vi "Double FFT Mesurament (Max Bin detection - Control - Windowing - LEO) test.vi"() -> ()   [LabVIEW 2014]
uses:
  <vilib>/Platform/TimedLoop/XDataNode/timing_clust.ctl
  <vilib>/Platform/TimedLoop/XDataNode/nitl_modes.ctl
  <vilib>/Platform/TimedLoop/XDataNode/wakeup.ctl
  <vilib>/rvi/Analysis/measure/FFT/simModelSupport/niFPGA FFT Streaming Sim Properties.ctl
  <vilib>/rvi/Analysis/measure/FFT/simModelSupport/niFPGA FFT Sim Stream Group Properties.ctl
  <vilib>/rvi/Analysis/measure/FFT/simModelSupport/niFPGA FFT Sim Types.ctl
  <vilib>/rvi/Analysis/measure/FFT/simModelSupport/niFpgaFFTSimArithmeticProperties.ctl
  <vilib>/rvi/Analysis/measure/FFT/simModelSupport/niFpgaFFTSimDfxp.ctl
  <vilib>/fxp/LVFixedPointQuantizationPolicyTypeDef.ctl
  <vilib>/rvi/Analysis/measure/FFT/XNode/niFpgaFFTButterflyDelays.ctl
  <vilib>/rvi/Emulation/niFpgaSctlEmulationGetInTimedLoop.vi
  <vilib>/rvi/Emulation/niFpgaEmulationReportErrorSimple.vi
  <vilib>/rvi/Emulation/niFpgaGetClockAttributes.vi
  <vilib>/rvi/Emulation/niFpgaCriticalErrorInLSC.vi
  <vilib>/rvi/Emulation/niFpgaEmulationIsFPGAContextNoSignature.vi
  <vilib>/rvi/errors/niFpgaSetErrorForExecOnDevCompSimple.vi
  <vilib>/rvi/eio/common/nirviEmuReportErrorAndStop.vi
  <vilib>/rvi/DataTransferAndStorage/Container/Common/niFpgaContainerGetUniqueNameForEmu.vi
  <vilib>/rvi/FIFO/Fifo_Resource/nirvififoEmulationSetSize.vi
  <vilib>/rvi/FIFO/Fifo_Resource/nirviFifoEmulationQueueMgr.vi
  <instcachedir>/0/nirviFifoEmulationQueueMgr_E5CAEC123FF24DC58D834DCA3CDAA9B5.lvgen/nirviFifoEmulationQueueMgr_E5CAEC123FF24DC58D834DCA3CDAA9B5_012.vi
  <vilib>/rvi/FIFO/Fifo_Resource/nirvififoEmulationCreateLock.vi
  <vilib>/rvi/Emulation/niFpgaProcessEmulError.vi
  <vilib>/rvi/FIFO/Fifo_Resource/nirvififoEmulationObtainLock.vi
  <vilib>/rvi/FIFO/Fifo_Resource/nirvififoEmulationReleaseLock.vi
  <vilib>/rvi/occurrence/nirviWaitOnOccurrenceBase.vi
  <vilib>/rvi/errors/nirviReportUnexpectedCaseInternalError.vi
  <vilib>/rvi/errors/nirviReportUnexpectedCaseInternalError (U32).vi
  <vilib>/rvi/Memory/Memory_Emulation/niFpgaMemoryEmulationCacheClearOnFirstRun.vi
  <vilib>/rvi/Memory/Memory_Emulation/nirvimemoryEmulationManagerCache_MakeExclusive.vi
  <vilib>/rvi/Memory/Memory_Emulation/niFpgaMemoryEmulationValidateCache.vi
  <vilib>/rvi/Memory/Memory_Emulation/nirvimemoryEmulationManagerCache_InsertValue.vi
  <vilib>/Utility/error.llb/Clear Errors.vi
  <vilib>/rvi/Memory/Memory_Emulation/nirvimemoryEmulationManagerCache_ReleaseExclusive.vi
  <vilib>/rvi/Memory/Memory_Emulation/nirvimemoryEmulationManagerCache_GetValue.vi
  <vilib>/rvi/Memory/Memory_Emulation/nirvimemoryEmulationManagerCache_SetValue.vi
  <vilib>/rvi/interface/RandomDataEmulation/niFpgaRandomDataHandleErrors.vi
  <instcachedir>/0/nirviFifoEmulationQueueMgr_E5CAEC123FF24DC58D834DCA3CDAA9B5.lvgen/nirviFifoEmulationQueueMgr_E5CAEC123FF24DC58D834DCA3CDAA9B5_010.vi
  <vilib>/rvi/FIFO/Fifo_Resource/nirvififoEmulationDetermineInputValidOut.vi
  <vilib>/rvi/Memory/Memory_Emulation/nirvimemoryFastEmulation.vi
  <vilib>/rvi/Memory/Memory_Emulation/nirvimemoryEmulation.vi
  <vilib>/rvi/Analysis/measure/FFT/simModelSupport/niFpgaFFTSimModelStreamingCore.vi
  <vilib>/rvi/eio/common/nirviEmuTemplateMethod_errors.vi
  <vilib>/Platform/TimedLoop/XDataNode/XDataNode.xnode
  <vilib>/rvi/DataTransferAndStorage/Container/XNode/niFpgaContainer.xnode
  <vilib>/rvi/FIFO/Fifo_Resource/nirvififoEmulationRead.vi
  <vilib>/rvi/DataTransferAndStorage/Register/Emulation/niFpgaRegisterEmulation.vi
  <vilib>/rvi/interface/RandomDataEmulation/nirviRandomDataFpgaReadWriteTemplate.vi
  <vilib>/rvi/FIFO/Fifo_Resource/nirvififoEmulationWrite.vi
  <vilib>/rvi/FIFO/Fifo_Resource/nirvififoEmulationGetNumberOfElementsToWrite.vi
  <vilib>/rvi/Analysis/measure/FFT/XNode/niFpgaFFT.xnode
  <vilib>/eio/EIOMethodNode/EIOMethodNode.xnode
  <vilib>/Platform/TimedLoop/XDataNode/XDNodeRunTimeDep.lvlib
panel:
  in  "first bin":i32=4
  in  "last bin":i32=251
  in  "lower limit 2":u32=682
  in  "lower limit 1":u32=57
  in  "upper limit 2":u32=1194
  in  "upper limit 1":u32=569
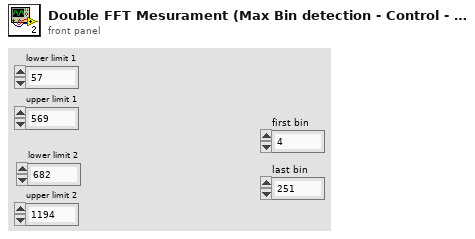
[diagram p1: front panel]
types:
  T1 = typedef "XDNodeRunTimeDep.lvlib/timing_clust.ctl" = cluster{"Expected End [f-1]":u64, "Actual End [f-1]":u64, "Finished Late? [f-1]":bool, "Expected End [i-1]":u64, "Actual End [i-1]":u64, "Finished Late? [i-1]":bool, "Expected Start [i]":u64, "Actual Start [i]":u64, "Expected Start [f]":u64, "Actual Start [f]":u64, "Source Name":string, "Structure Name":string, "Period":i64, "Deadline":i64, "Offset":i64, "Start":i64, "Priority":i32, "Timeout":i32, "Mode":T2, "Wakeup Reason":T3, "Error":errorcluster, "Source Type":string, "Secondary Source Type":string, "Global End Time":u64, "Global Start Time":u64, "Frame Duration":u64, "Iteration Duration":u64, "Assigned CPU":i32, "I/O Scan Engine Mode":u32}
  T2 = typedef "XDNodeRunTimeDep.lvlib/nitl_modes.ctl" = enum32{"No Change", "Process missed periods, maintain original phase", "Discard missed periods, maintain original phase", "Process missed periods, ignore original phase", "Discard missed periods, ignore original phase"}
  T3 = typedef "XDNodeRunTimeDep.lvlib/wakeup.ctl" = enum32{"Normal", "Aborted", "Asynchronous wakeup", "Timing source error", "Timed loop error", "Timeout"}
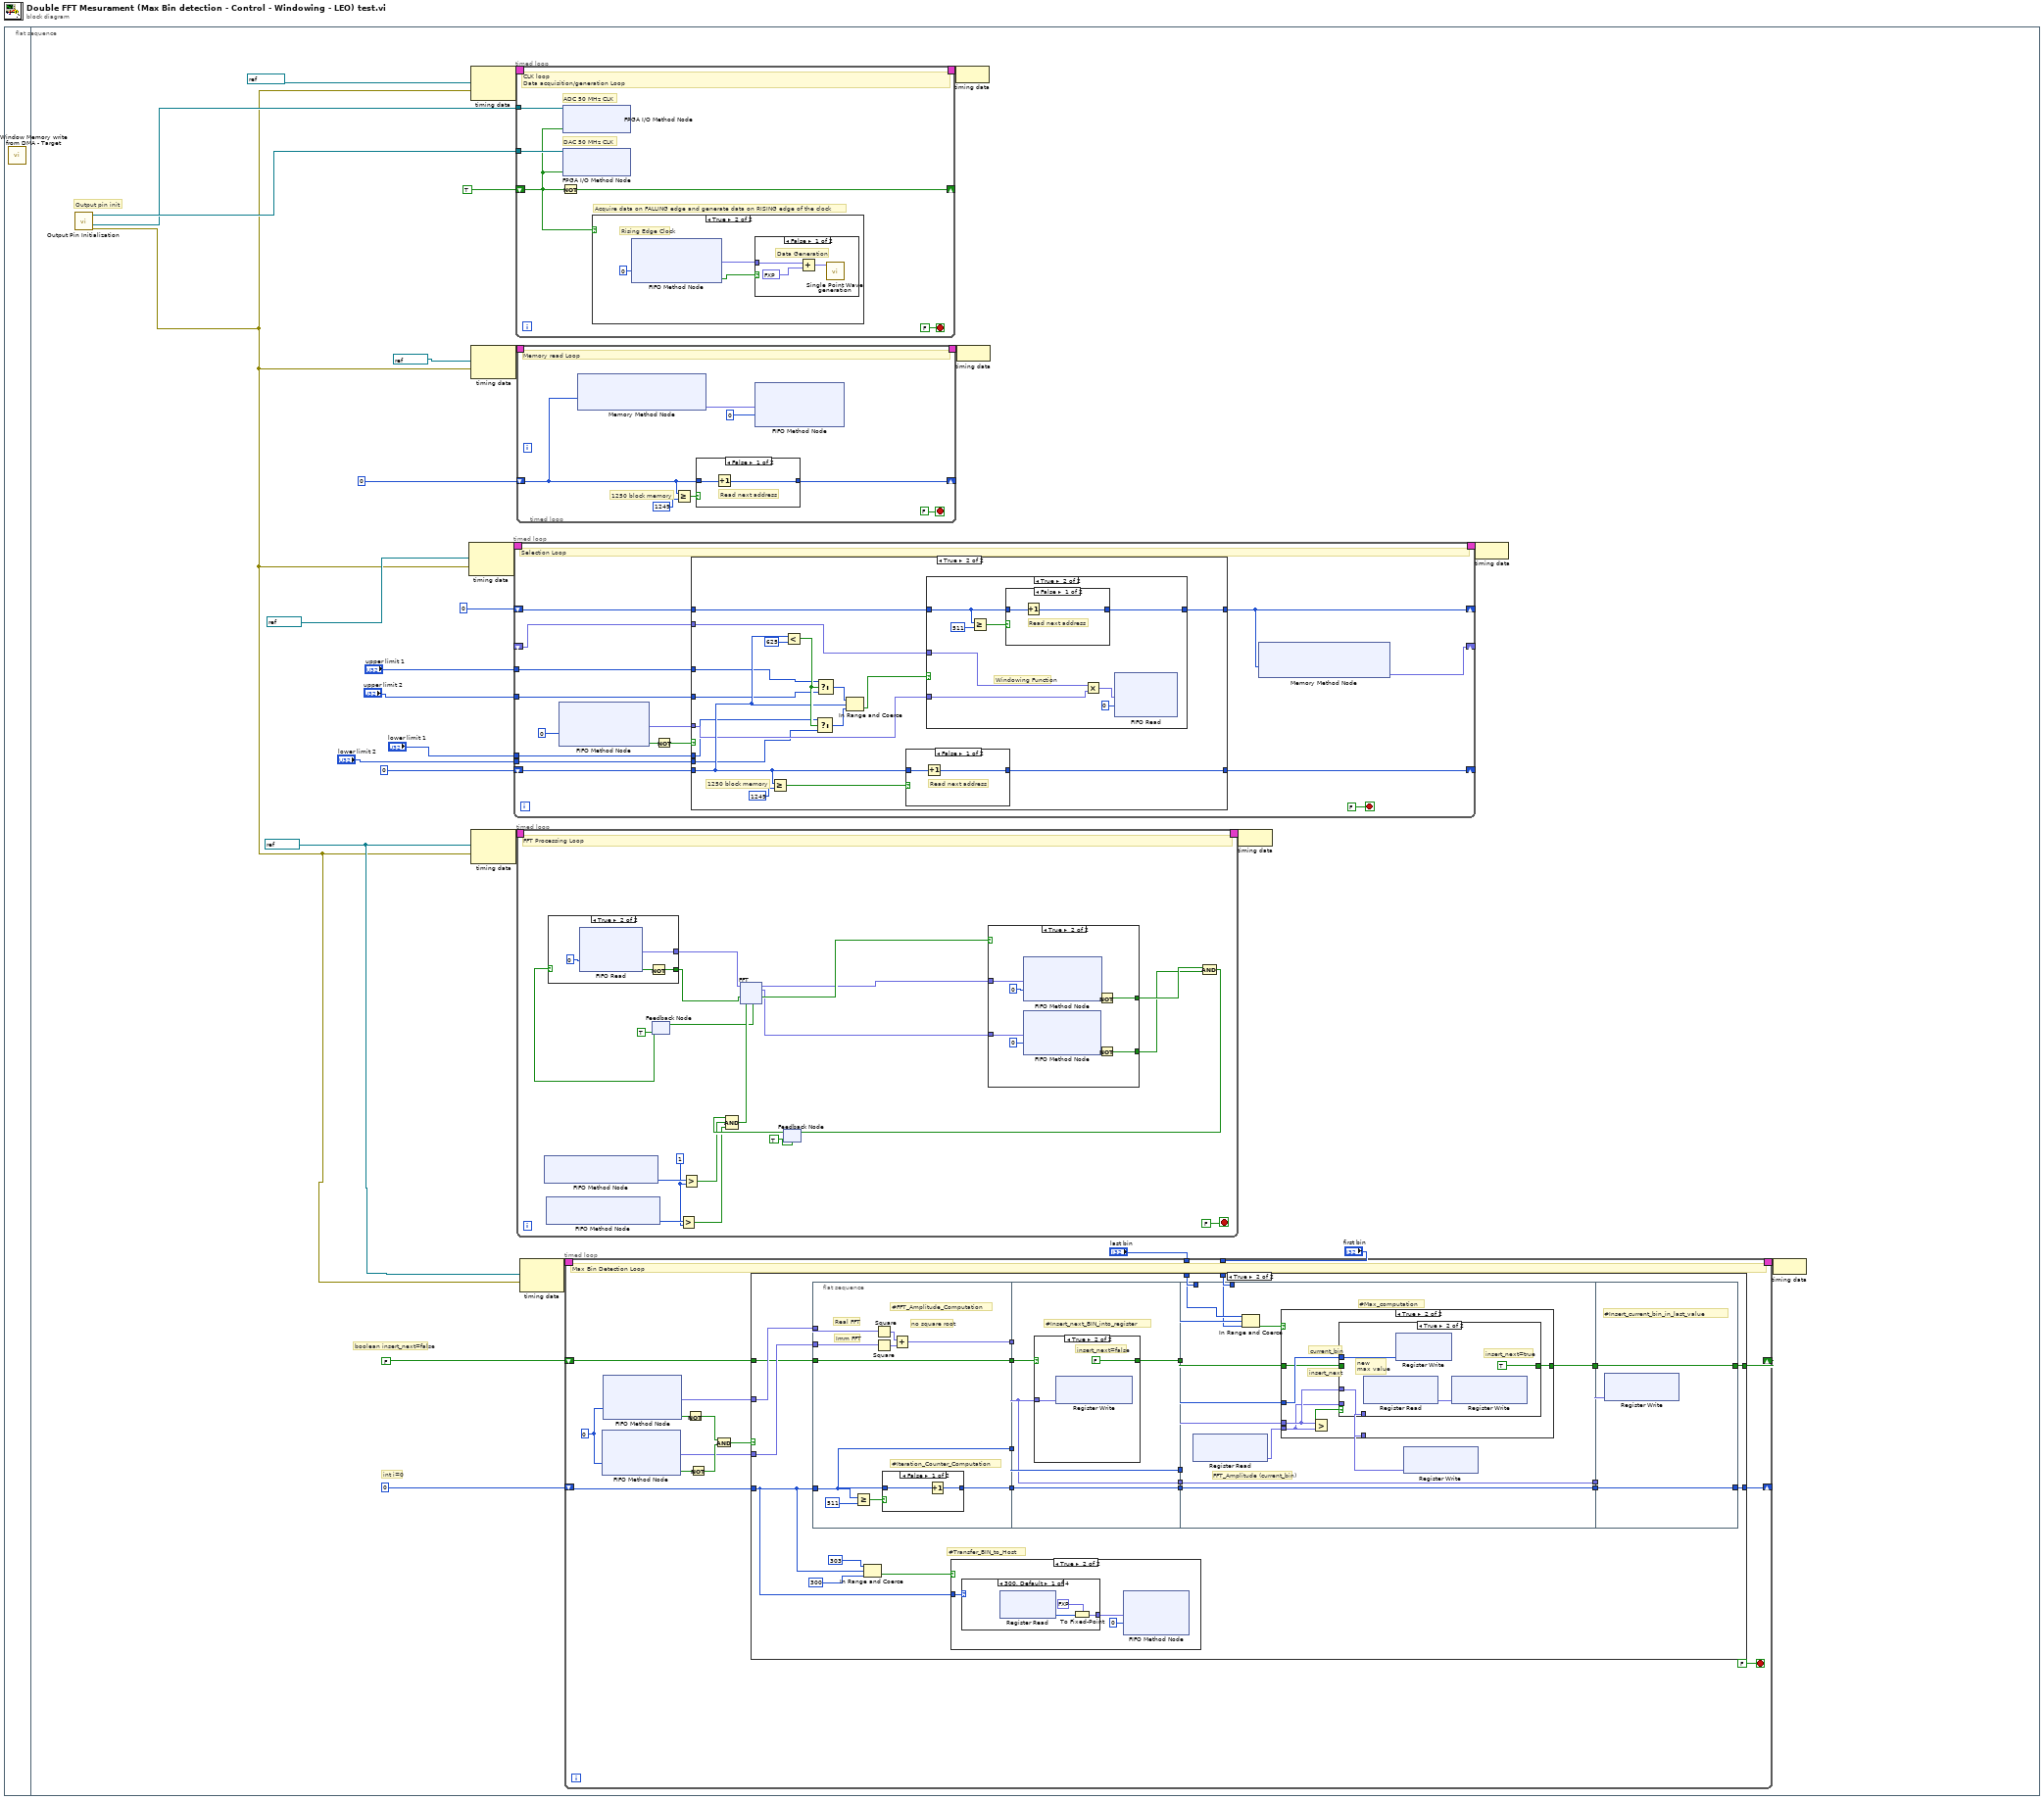
[diagram p0: block diagram]
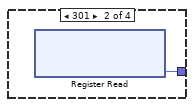
[diagram p4: hidden frame]
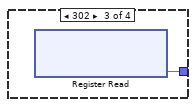
[diagram p5: hidden frame]
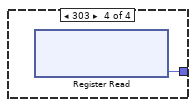
[diagram p6: hidden frame]
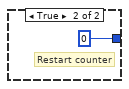
[diagram p7: hidden frame]
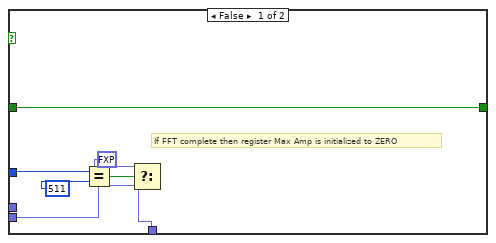
[diagram p9: hidden frame]
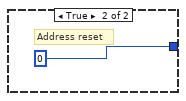
[diagram p13: hidden frame]
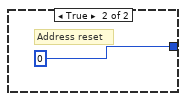
[diagram p14: hidden frame]
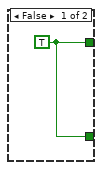
[diagram p15: hidden frame]
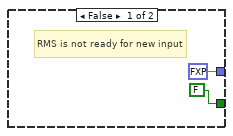
[diagram p16: hidden frame]
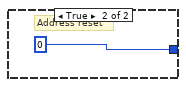
[diagram p17: hidden frame]
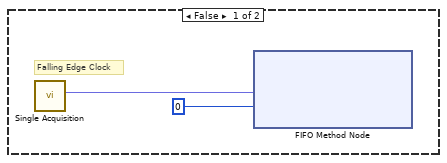
[diagram p18: hidden frame]
diagram:
  n1 = flat-sequence {
    frame #0 {
      n2 = call "Window Memory write from DMA - Target.vi"() -> ()  [unwired: 12 in]
    }
    frame #1 {
      w9 = refnum<k21> "50MHz" ("Source Name")
      # "int i=0"
      # "boolean insert_next=false"
      # "Output pin init"
      n3 = call "Output Pin Initialization.vi"() -> ("error out"=w8:errorcluster, "I/O Out Clock DAC (pin16)"=w14:refnum<k21>, "I/O Out Clock ADC (pin17)"=w15:refnum<k21>)  [unwired: 8 in]
      n4 = node-c288(refnum<k21> "50MHz" ("Source Name"), w8) -> (w23:T1)
      n5 = node-c288(refnum<k21> "100MHz" ("Source Name"), w8) -> (w29:T1)
      n6 = node-c288(refnum<k21> "50MHz" ("Source Name"), w8) -> (w27:T1)
      n7 = node-c288(w9, w8) -> (w25:T1)
      n8 = timed-loop {
        timing: w23 -> [_]
        timing-out: [_] -> w22
        shift-right: [w152] -> _
        shift-left: u32 0 -> [w151]
        tunnel: "upper limit 1" -> [w146]
        tunnel: "upper limit 2" -> [w145]
        tunnel: "lower limit 1" -> [w144]
        tunnel: "lower limit 2" -> [w143]
        shift-right: [w139] -> _
        shift-left: u32 0 -> [w142]
        shift-right: [w140] -> _
        shift-left: _ -> [w141]
        stop <- FALSE stop-if-true
        # "Selection Loop"
        n9 = xnode ("FIFO Method Node")("Timeout"=0) -> ("Element"=w148:fxp<+/-,12,12>, "Timed Out?"=w149:bool)  [unwired: 1 in, 1 out]
        n10 = Not(x=w149) -> (.not. x?=w150:bool)
        n11 = case shown="True" w150 {
          tunnel: [w155 w170] -> w152
          tunnel: w151 -> [w155 w165]
          tunnel: w148 -> [_ w163]
          tunnel: w146 -> [_ w162]
          tunnel: w145 -> [_ w161]
          tunnel: w144 -> [_ w160]
          tunnel: w143 -> [_ w159]
          tunnel: w142 -> [w154 w156]
          tunnel: [w154 w158] -> w139
          tunnel: w141 -> [_ w157]
          frame False {
          }
          frame True {
            # "1250 block memory"
            n12 = Greater Or Equal?(x=w165, y=u32 1249) -> (x >= y?=w171:bool)
            n13 = Less?(x=w165, y=u32 625) -> (x < y?=w166:bool)
            n14 = Select(t=w160, s=w166, f=w159) -> (s? t:f=w168:u32)
            n15 = Select(t=w162, s=w166, f=w161) -> (s? t:f=w169:u32)
            n16 = In Range and Coerce(upper limit=w169, x=w165, lower limit=w168) -> (In Range?=w164:bool)  [unwired: 1 out]
            n17 = case shown="False" w171 {
              tunnel: w165 -> [w186 _]
              tunnel: [w185 u32 0] -> w170
              frame False {
                # "Read next address"
                n18 = Increment(x=w186) -> (x+1=w185:u32)
              }
              frame True {
                # "Address reset"
              }
            }
            n19 = case shown="True" w164 {
              tunnel: w163 -> [_ w180]
              tunnel: w156 -> [w173 w176]
              tunnel: [w173 w178] -> w158
              tunnel: w157 -> [_ w174]
              frame False {
              }
              frame True {
                # "Windowing Function"
                n20 = Greater Or Equal?(x=w176, y=u32 511) -> (x >= y?=w177:bool)
                n21 = case shown="False" w177 {
                  tunnel: w176 -> [w183 _]
                  tunnel: [w182 u32 0] -> w178
                  frame False {
                    # "Read next address"
                    n22 = Increment(x=w183) -> (x+1=w182:u32)
                  }
                  frame True {
                    # "Address reset"
                  }
                }
                n23 = Multiply(x=w174, y=w180) -> (x*y=w179:fxp<+/-,12,12>)
                n24 = xnode ("FIFO Read")("Element"=w179, "Timeout"=0) -> ()  [unwired: 1 in, 2 out]
              }
            }
          }
        }
        n25 = xnode ("Memory Method Node")("Address"=w139) -> ("Data"=w140:fxp<+,8,1>)  [unwired: 1 in, 1 out]
      }
      n26 = timed-loop {
        timing: w29 -> [_]
        timing-out: [_] -> w28
        shift-right: [w282] -> _
        shift-left: TRUE -> [w280]
        tunnel: w14 -> [w284]
        tunnel: w15 -> [w281]
        stop <- FALSE stop-if-true
        # "DAC 50 MHz CLK"
        # "Acquire data on FALLING edge and generate data on RISING edge of the clock"
        # "ADC 50 MHz CLK"
        # "CLK loop\nData acquisition/generation Loop"
        n27 = Not(x=w280) -> (.not. x?=w282:bool)
        n28 = xnode "FPGA I/O Method Node"("FPGA I/O In"=w284, "Data"=w280) -> ()  [unwired: 1 out]
        n29 = xnode "FPGA I/O Method Node"("FPGA I/O In"=w281, "Data"=w280) -> ()  [unwired: 1 out]
        n30 = case shown="True" w280 {
          frame False {
            # "Falling Edge Clock"
            n31 = call "Single Acquisition.vi"() -> ("Out"=w286:fxp<+/-,12,12>)  [unwired: 10 in, 1 out]
            n32 = xnode ("FIFO Method Node")("Element"=w286, "Timeout"=0) -> ()  [unwired: 1 in, 2 out]
          }
          frame True {
            # "Rising Edge Clock"
            n33 = xnode ("FIFO Method Node")("Timeout"=0) -> ("Element"=w287:fxp<+/-,12,12>, "Timed Out?"=w288:bool)  [unwired: 1 in, 1 out]
            n34 = case shown="False" w288 {
              tunnel: w287 -> [w292 _]
              frame False {
                # "Data Generation"
                n35 = Add(x=w292, y=fxp<+,12,12> 2048.0) -> (x+y=w290:fxp<+/-,14,14>)
                n36 = call "Single Point Wave generation.vi"("Data To Write"=w290) -> ()  [unwired: 10 in, 1 out]
              }
              frame True {
                # "FPGA memory slow"
              }
            }
          }
        }
      }
      n37 = timed-loop {
        timing: w27 -> [_]
        timing-out: [_] -> w26
        shift-right: [w267] -> _
        shift-left: u32 0 -> [w265]
        stop <- FALSE stop-if-true
        # "1250 block memory"
        # "Memory read Loop"
        n38 = xnode ("Memory Method Node")("Address"=w265) -> ("Data"=w264:fxp<+/-,12,12>)  [unwired: 1 in, 1 out]
        n39 = Greater Or Equal?(x=w265, y=u32 1249) -> (x >= y?=w268:bool)
        n40 = case shown="False" w268 {
          tunnel: w265 -> [w271 _]
          tunnel: [w270 u32 0] -> w267
          frame False {
            # "Read next address"
            n41 = Increment(x=w271) -> (x+1=w270:u32)
          }
          frame True {
            # "Address reset"
          }
        }
        n42 = xnode ("FIFO Method Node")("Element"=w264, "Timeout"=0) -> ()  [unwired: 1 in, 2 out]
      }
      n43 = timed-loop {
        timing: w25 -> [_]
        timing-out: [_] -> w24
        stop <- FALSE stop-if-true
        w197 = u32 1 ("y")
        # "FFT Processing Loop"
        n44 = xnode ("FIFO Method Node")() -> ("Number of Elements to Write"=w199:u32)  [unwired: 1 in, 1 out]
        n45 = xnode ("FIFO Method Node")() -> ("Number of Elements to Write"=w198:u32)  [unwired: 1 in, 1 out]
        n46 = feedback #1(TRUE ("ready for input")) -> (w214:bool)
        n47 = case shown="True" w214 {
          tunnel: [FALSE w255] -> w208
          tunnel: [fxp<+/-,12,12> 0.0 ("Element") w252] -> w209
          frame False {
            # "RMS is not ready for new input"
          }
          frame True {
            n48 = xnode ("FIFO Read")("Timeout"=0) -> ("Element"=w252:fxp<+/-,12,12>, "Timed Out?"=w254:bool)  [unwired: 1 in, 1 out]
            n49 = Not(x=w254) -> (.not. x?=w255:bool)
          }
        }
        n50 = Greater?(x=w198, y=w197) -> (0:w195:bool)
        n51 = Greater?(x=w199, y=w197) -> (0:w196:bool)
        n52 = feedback #2(TRUE) -> (w210:bool)
        n53 = Compound Arithmetic op=AND(w210, w196, w195) -> (w207:bool)
        n54 = xnode "FFT"("real data in"=w209, "input valid"=w208, "ready for output"=w207) -> ("ready for input"=w206:bool, "real data out"=w204:fxp<+/-,22,22>, "imaginary data out"=w203:fxp<+/-,22,22>, "output valid"=w205:bool)  [unwired: 2 in, 1 out]
        n55 = feedback-in #1(w206) -> ()
        n56 = case shown="True" w205 {
          tunnel: w204 -> [_ w249]
          tunnel: w203 -> [_ w248]
          tunnel: [w241 w247] -> w202
          tunnel: [w241 w246] -> w201
          frame False {
            w241 = TRUE
          }
          frame True {
            n57 = xnode ("FIFO Method Node")("Element"=w249, "Timeout"=0) -> ("Timed Out?"=w242:bool)  [unwired: 1 in, 1 out]
            n58 = xnode ("FIFO Method Node")("Element"=w248, "Timeout"=0) -> ("Timed Out?"=w243:bool)  [unwired: 1 in, 1 out]
            n59 = Not(x=w242) -> (.not. x?=w247:bool)
            n60 = Not(x=w243) -> (.not. x?=w246:bool)
          }
        }
        n61 = Compound Arithmetic op=AND(w202, w201) -> (w200:bool)
        n62 = feedback-in #2(w200) -> ()
      }
      n63 = node-c288(w9, w8) -> (w21:T1)
      n64 = timed-loop {
        shift-right: [w35] -> _
        shift-left: 0 ("Timeout") -> [w36]
        shift-right: [w33] -> _
        shift-left: FALSE -> [w34]
        timing: w21 -> [_]
        timing-out: [_] -> w20
        tunnel: "last bin" -> [w31]
        tunnel: "first bin" -> [w30]
        stop <- FALSE stop-if-true
        w44 = 0 ("Timeout")
        # "Max Bin Detection Loop"
        n65 = xnode ("FIFO Method Node")("Timeout"=w44) -> ("Element"=w37:fxp<+/-,22,22>, "Timed Out?"=w42:bool)  [unwired: 1 in, 1 out]
        n66 = xnode ("FIFO Method Node")("Timeout"=w44) -> ("Element"=w38:fxp<+/-,22,22>, "Timed Out?"=w43:bool)  [unwired: 1 in, 1 out]
        n67 = Not(x=w43) -> (.not. x?=w41:bool)
        n68 = Not(x=w42) -> (.not. x?=w40:bool)
        n69 = And(x=w41, y=w40) -> (x .and. y?=w39:bool)
        n70 = case shown="True" w39 {
          tunnel: w38 -> [_ w68]
          tunnel: w37 -> [_ w67]
          tunnel: w36 -> [w46 w47]
          tunnel: [w46 w53] -> w35
          tunnel: w34 -> [w45 w60]
          tunnel: [w45 w55] -> w33
          tunnel: w31 -> [_ w52]
          tunnel: w30 -> [_ w51]
          frame False {
            # "Data are NOT ready in Target Real FFT and Target Imm FFT FIFOs"
          }
          frame True {
            # "#Transfer_BIN_to_Host"
            n71 = flat-sequence {
              tunnel: w68 -> [w84]
              tunnel: w67 -> [w85]
              tunnel: [w83] -> w66
              tunnel: w47 -> [w78]
              tunnel: [w82] -> w65
              tunnel: [w78] -> w62
              tunnel: [w79] -> w61
              tunnel: w60 -> [w79]
              tunnel: w66 -> [w92]
              tunnel: w65 -> [w95]
              tunnel: [w95] -> w64
              tunnel: w62 -> [w93]
              tunnel: w61 -> [w94]
              tunnel: [w93] -> w59
              tunnel: [w92] -> w58
              tunnel: [w91] -> w57
              tunnel: w64 -> [w108]
              tunnel: [w108] -> w63
              tunnel: w59 -> [w103]
              tunnel: w58 -> [w105]
              tunnel: w57 -> [w106]
              tunnel: [w105] -> w56
              tunnel: [w104] -> w54
              tunnel: w52 -> [w100]
              tunnel: w51 -> [w99]
              tunnel: w63 -> [w129]
              tunnel: w56 -> [w131]
              tunnel: w54 -> [w130]
              tunnel: [w130] -> w55
              tunnel: [w129] -> w53
              frame #0 {
                # "no square root"
                # "#Iteration_Counter_Computation"
                # "#FFT_Amplitude_Computation"
                # "Imm FFT"
                # "Real FFT"
                n72 = Greater Or Equal?(x=w78, y=511) -> (x >= y?=w80:bool)
                n73 = Square(x=w84) -> (x^2=w87:fxp<+,43,43>)
                n74 = Square(x=w85) -> (x^2=w86:fxp<+,43,43>)
                n75 = case shown="False" w80 {
                  tunnel: w78 -> [w88 _]
                  tunnel: [w89 0 ("Timeout")] -> w82
                  frame False {
                    n76 = Increment(x=w88) -> (x+1=w89:i32)
                  }
                  frame True {
                    # "Restart counter"
                  }
                }
                n77 = Add(x=w87, y=w86) -> (x+y=w83:fxp<+,44,44>)
              }
              frame #1 {
                # "#Insert_next_BIN_into_register"
                n78 = case shown="True" w94 {
                  selector: w94 -> [w96 _]
                  tunnel: [w96 FALSE] -> w91
                  tunnel: w92 -> [_ w97]
                  frame False {
                  }
                  frame True {
                    # "insert_next=false"
                    n79 = xnode ("Register Write")("Data"=w97) -> ()  [unwired: 1 in, 1 out]
                  }
                }
              }
              frame #2 {
                # "FFT_Amplitude (current_bin)"
                # "#Max_computation"
                n80 = xnode ("Register Read")() -> ("Data"=w102:fxp<+,44,44>)  [unwired: 1 in, 1 out]
                n81 = In Range and Coerce(upper limit=w100, x=w103, lower limit=w99) -> (In Range?=w107:bool)  [unwired: 1 out]
                n82 = case shown="True" w107 {
                  tunnel: w105 -> [_ w121]
                  tunnel: w103 -> [w113 w120]
                  tunnel: w106 -> [w115 w119]
                  tunnel: [w115 w118] -> w104
                  tunnel: w102 -> [w111 w116]
                  tunnel: [w109 w117] -> w101
                  frame False {
                    # "If FFT complete then register Max Amp is initialized to ZERO"
                    n83 = Equal?(x=w113, y=511) -> (x = y?=w114:bool)
                    n84 = Select(t=fxp<+,44,44> 0.0, s=w114, f=w111) -> (s? t:f=w109:fxp<+,44,44>)
                  }
                  frame True {
                    # "insert_next"
                    # "current_bin"
                    n85 = Greater?(x=w121, y=w116) -> (0:w122:bool)
                    n86 = case shown="True" w122 {
                      tunnel: w121 -> [_ w125]
                      tunnel: w120 -> [_ w128]
                      tunnel: w119 -> [w124 _]
                      tunnel: [w124 TRUE] -> w118
                      tunnel: [w123 w125] -> w117
                      tunnel: w116 -> [w123 _]
                      frame False {
                        # "Old value is re-written"
                      }
                      frame True {
                        # "new\nmax value"
                        # "insert_next=true"
                        n87 = xnode ("Register Read")() -> ("Data"=w126:fxp<+,44,44>)  [unwired: 1 in, 1 out]
                        n88 = xnode ("Register Write")("Data"=w128) -> ()  [unwired: 1 in, 1 out]
                        n89 = xnode ("Register Write")("Data"=w126) -> ()  [unwired: 1 in, 1 out]
                      }
                    }
                  }
                }
                n90 = xnode ("Register Write")("Data"=w101) -> ()  [unwired: 1 in, 1 out]
              }
              frame #3 {
                # "#Insert_current_bin_in_last_value"
                n91 = xnode ("Register Write")("Data"=w131) -> ()  [unwired: 1 in, 1 out]
              }
            }
            n92 = In Range and Coerce(upper limit=303 ("y"), x=w47, lower limit=300) -> (In Range?=w50:bool)  [unwired: 1 out]
            n93 = case shown="True" w50 {
              tunnel: w47 -> [_ w71]
              frame False {
                # "FFT Comp is NOT finished"
              }
              frame True {
                n94 = case shown="300, Default" w71 {
                  tunnel: [w72 w75 w76 w77] -> w70
                  frame 300, Default {
                    n95 = xnode ("Register Read")() -> ("Data"=w73:i32)  [unwired: 1 in, 1 out]
                    n96 = To Fixed-Point(fixed-point type=fxp<+,44,44> 0.0 ("Data"), number=w73) -> (fixed-point=w72:fxp<+,44,44>)
                  }
                  frame 301 {
                    n97 = xnode ("Register Read")() -> ("Data"=w75:fxp<+,44,44>)  [unwired: 1 in, 1 out]
                  }
                  frame 302 {
                    n98 = xnode ("Register Read")() -> ("Data"=w76:fxp<+,44,44>)  [unwired: 1 in, 1 out]
                  }
                  frame 303 {
                    n99 = xnode ("Register Read")() -> ("Data"=w77:fxp<+,44,44>)  [unwired: 1 in, 1 out]
                  }
                }
                n100 = xnode ("FIFO Method Node")("Element"=w70, "Timeout"=0) -> ()  [unwired: 1 in, 2 out]
              }
            }
          }
        }
      }
      n101 = node-c288(w28) -> ()
      n102 = node-c288(w26) -> ()
      n103 = node-c288(w24) -> ()
      n104 = node-c288(w22) -> ()
      n105 = node-c288(w20) -> ()
    }
  }
